vi "Autonomous Independent.vi"() -> ()   [LabVIEW 2018]
doc: "This VI is called when autonomous begins, and will automatically be terminated when autonomous ends. You can carry out timed or sensor driven robot movement independently without needing to return to the caller."
uses:
  <vilib>/Rock Robotics/WPI/DriverStation/WPI_DriverStationDerivedRobotMode.ctl
  <vilib>/Rock Robotics/Network Tables/NT Read String.vi
  Robot Global Data.vi
panel:
  in  "Call Context":T1
  out "Potentiometer":dbl
  out "Yaw":dbl
  out "Right Motor Speed":dbl
  out "Left Motor Speed":dbl
  # "Be sure to right-click and choose Data Operations>>Make Current Value default if you want to save the array values with the VI"
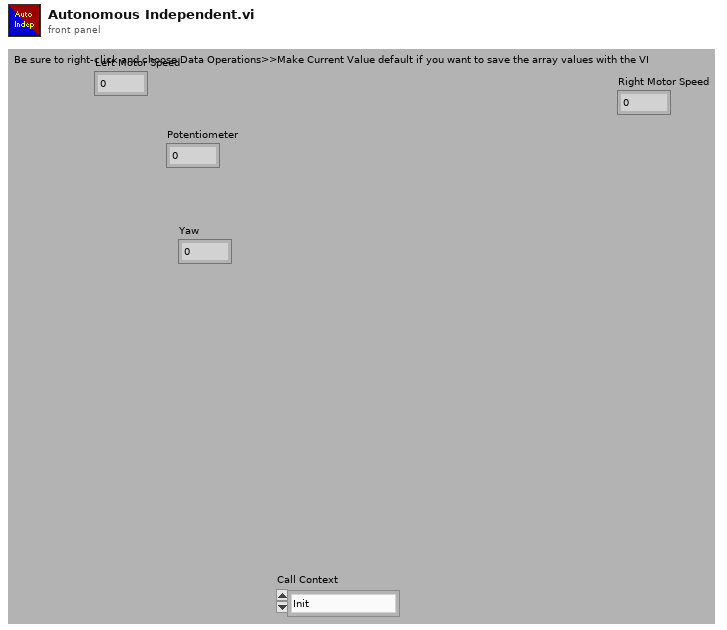
[diagram p1: front panel]
types:
  T1 = typedef "WPI_DriverStationDerivedRobotMode.ctl" = enum16{"Init", "Execute", "Stop"}
  T2 = typedef "WPI_JoystickDevRef.ctl" = cluster{"Device":T3}
  T3 = typedef "WPI_JoystickDeviceEnum.ctl" = enum16{"USB 0", "USB 1", "USB 2", "USB 3", "USB 4", "USB 5"}
  T4 = cluster{"Axes":dbl[], "Buttons":bool[], "POVs":i16[]}
  T5 = cluster{"Yaw":dbl, "Roll":dbl, "Pitch":dbl, "Heading":dbl, "Fused Heading":dbl}
  T6 = typedef "WPI_PotentiometerDevRef.ctl" = cluster{"DevStatus":errorcluster, "Analog Channel":T7, "Invert Output":bool}
  T7 = typedef "FPGA_AIChannel.ctl" = enum8{"AI 0", "AI 1", "AI 2", "AI 3", "AI MXP 0", "AI MXP 1", "AI MXP 2", "AI MXP 3", "Invalid"}
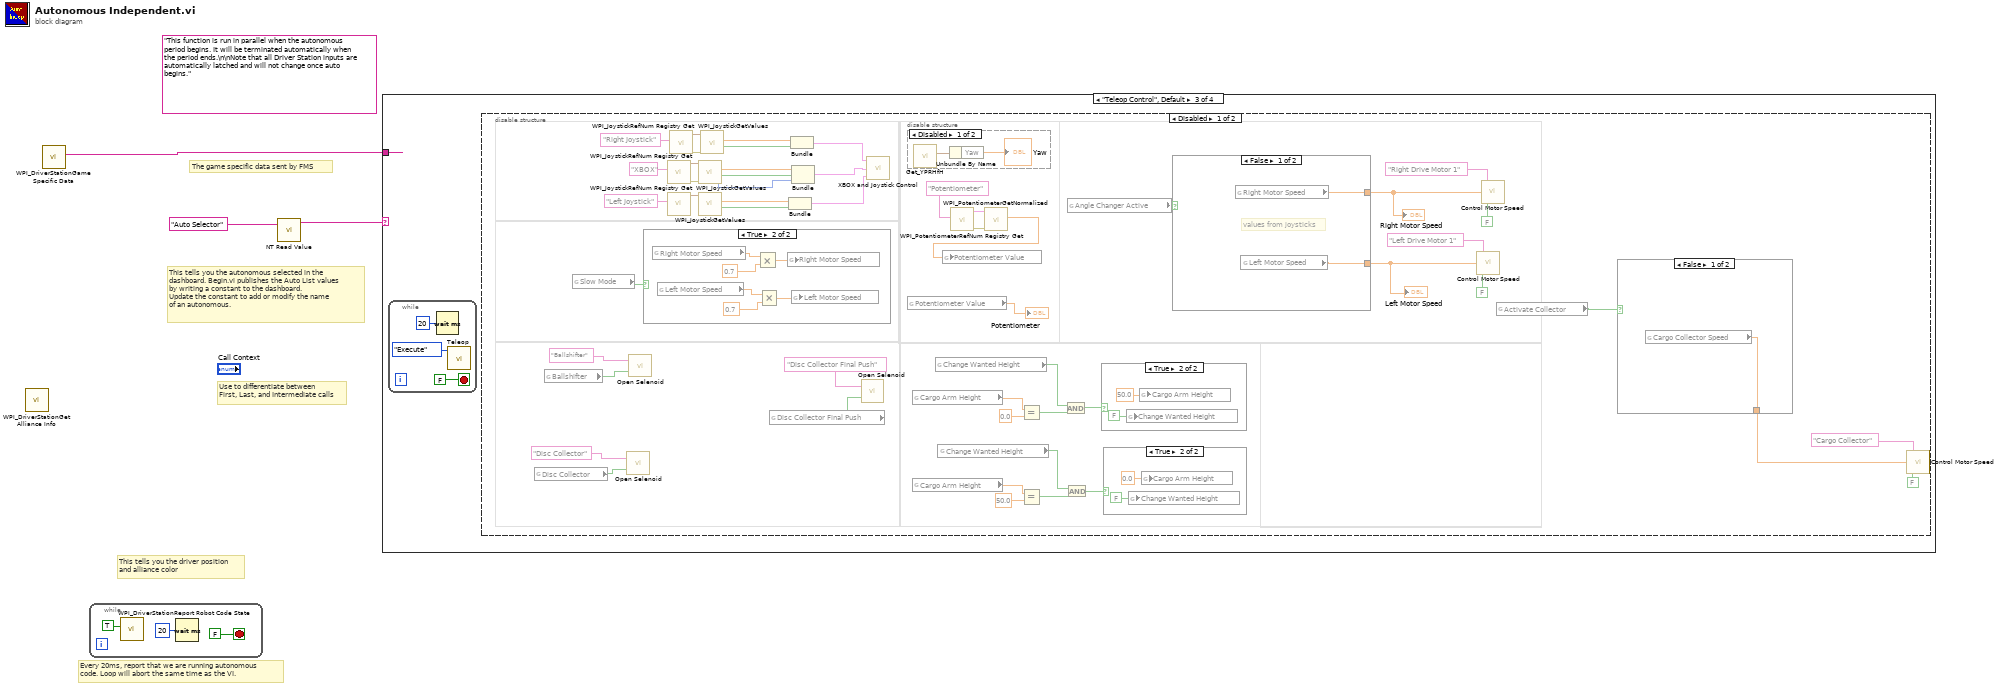
[diagram p0: block diagram]
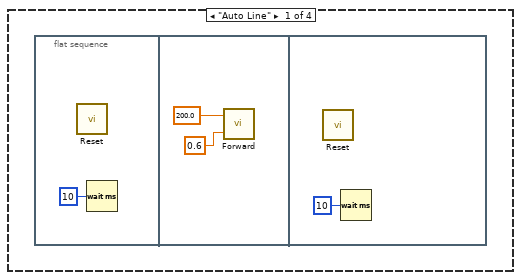
[diagram p2: hidden frame]
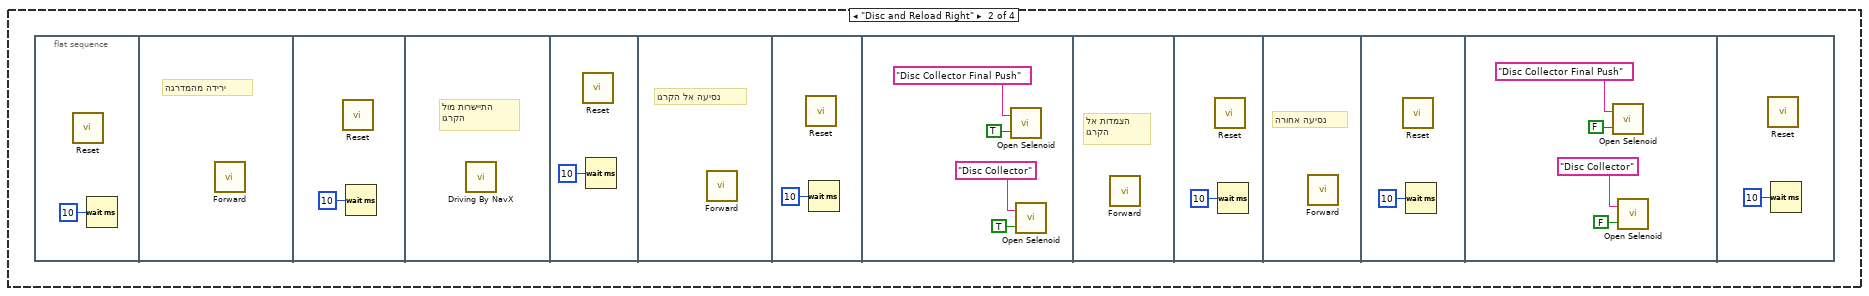
[diagram p3: hidden frame]
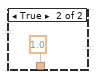
[diagram p4: hidden frame]
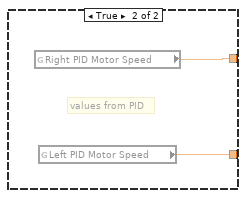
[diagram p6: hidden frame]
diagram:
  (unwired) "This function is run in parallel when the autonomous period begins. It will be terminated automatically when the period ends.\n\nNote that all Driver Station inputs are automatically latched and will not change once auto begins."
  # "Use to differentiate between\nFirst, Last, and Intermediate calls"
  # "The game specific data sent by FMS"
  # "This tells you the autonomous selected in the \ndashboard. Begin.vi publishes the Auto List values\nby writing a constant to the dashboard.\nUpdate the constant to add or modify the name\nof an autonomous."
  # "Every 20ms, report that we are running autonomous\ncode. Loop will abort the same time as the VI."
  # "This tells you the driver position\nand alliance color"
  n1 = call <vilib>:"WPI_DriverStationGet Alliance Info.vi"() -> ()  [unwired: 12 out]
  n2 = call <vilib>:"WPI_DriverStationGame Specific Data.vi"() -> ("Game Specific Data"=w1:string)  [unwired: 11 in]
  n3 = while {
    stop <- FALSE stop-if-true
    n4 = call <vilib>:"WPI_DriverStationReport Robot Code State.vi"("Autonomous"=TRUE) -> ()  [unwired: 10 in, 1 out]
    n5 = Wait (ms)(milliseconds to wait=u32 20) -> ()  [unwired: 1 out]
  }
  n6 = call-poly <vilib>:"NT Read Value.vi"("Name"="Auto Selector") -> ("String"=w2:string)  [unwired: 9 in, 1 out]
  n7 = case shown="\"Teleop Control\", Default" w2 {
    tunnel: w1 -> [_ _ _ _]
    frame "Auto Line" {
      n8 = flat-sequence {
        frame #0 {
          n9 = call "Reset.vi"() -> ()  [unwired: 1 in]
          n10 = Wait (ms)(milliseconds to wait=u32 10) -> ()  [unwired: 1 out]
        }
        frame #1 {
          n11 = call "Forward.vi"("Speed"=0.6, "Driving Distance"=200.0) -> ()  [unwired: 1 in]
        }
        frame #2 {
          n12 = call "Reset.vi"() -> ()  [unwired: 1 in]
          n13 = Wait (ms)(milliseconds to wait=u32 10) -> ()  [unwired: 1 out]
        }
      }
    }
    frame "Disc and Reload Right" {
      n14 = flat-sequence {
        frame #0 {
          n15 = call "Reset.vi"() -> ()  [unwired: 1 in]
          n16 = Wait (ms)(milliseconds to wait=u32 10) -> ()  [unwired: 1 out]
        }
        frame #1 {
          # "ירידה מהמדרגה"
          n17 = call "Forward.vi"() -> ()  [unwired: 3 in]
        }
        frame #2 {
          n18 = call "Reset.vi"() -> ()  [unwired: 1 in]
          n19 = Wait (ms)(milliseconds to wait=u32 10) -> ()  [unwired: 1 out]
        }
        frame #3 {
          # "התיישרות מול\nהקרגו"
          n20 = call "Driving By NavX.vi"() -> ()  [unwired: 4 in]
        }
        frame #4 {
          n21 = call "Reset.vi"() -> ()  [unwired: 1 in]
          n22 = Wait (ms)(milliseconds to wait=u32 10) -> ()  [unwired: 1 out]
        }
        frame #5 {
          # "נסיעה אל הקרגו"
          n23 = call "Forward.vi"() -> ()  [unwired: 3 in]
        }
        frame #6 {
          n24 = call "Reset.vi"() -> ()  [unwired: 1 in]
          n25 = Wait (ms)(milliseconds to wait=u32 10) -> ()  [unwired: 1 out]
        }
        frame #7 {
          n26 = call "Open Selenoid.vi"("Enable"=TRUE, "Selenoid Name"="Disc Collector Final Push") -> ()  [unwired: 1 in]
          n27 = call "Open Selenoid.vi"("Enable"=TRUE, "Selenoid Name"="Disc Collector") -> ()  [unwired: 1 in]
        }
        frame #8 {
          # "הצמדות אל\nהקרגו"
          n28 = call "Forward.vi"() -> ()  [unwired: 3 in]
        }
        frame #9 {
          n29 = call "Reset.vi"() -> ()  [unwired: 1 in]
          n30 = Wait (ms)(milliseconds to wait=u32 10) -> ()  [unwired: 1 out]
        }
        frame #10 {
          # "נסיעה אחורה"
          n31 = call "Forward.vi"() -> ()  [unwired: 3 in]
        }
        frame #11 {
          n32 = call "Reset.vi"() -> ()  [unwired: 1 in]
          n33 = Wait (ms)(milliseconds to wait=u32 10) -> ()  [unwired: 1 out]
        }
        frame #12 {
          n34 = call "Open Selenoid.vi"("Enable"=FALSE, "Selenoid Name"="Disc Collector Final Push") -> ()  [unwired: 1 in]
          n35 = call "Open Selenoid.vi"("Enable"=FALSE, "Selenoid Name"="Disc Collector") -> ()  [unwired: 1 in]
        }
        frame #13 {
          n36 = call "Reset.vi"() -> ()  [unwired: 1 in]
          n37 = Wait (ms)(milliseconds to wait=u32 10) -> ()  [unwired: 1 out]
        }
      }
    }
    frame "Teleop Control", Default {
      n38 = while {
        stop <- FALSE stop-if-true
        n39 = Wait (ms)(milliseconds to wait=u32 20) -> ()  [unwired: 1 out]
        n40 = call "Teleop.vi"("Call Context"=WPI_DriverStationDerivedRobotMode."Execute") -> ()  [unwired: 2 in, 9 out]
      }
      n41 = disable-structure shown="Disabled" {
        frame Disabled {
          n42 = global read "Robot Global Data.vi" "Disc Collector"() -> (w58:bool)
          n43 = global read "Robot Global Data.vi" "Ballshifter"() -> (w60:bool)
          n44 = global read "Robot Global Data.vi" "Slow Mode"() -> (w41:bool)
          n45 = call "Open Selenoid.vi"("Enable"=w58, "Selenoid Name"="Disc Collector") -> ()  [unwired: 1 in]
          n46 = call "Open Selenoid.vi"("Enable"=w60, "Selenoid Name"="Ballshifter") -> ()  [unwired: 1 in]
          n47 = case shown="True" w41 {
            frame False {
            }
            frame True {
              n48 = global read "Robot Global Data.vi" "Right Motor Speed"() -> (w92:dbl)
              n49 = global read "Robot Global Data.vi" "Left Motor Speed"() -> (w89:dbl)
              n50 = Multiply(x=w92, y=0.7) -> (x*y=w91:dbl)
              n51 = Multiply(x=w89, y=0.7) -> (x*y=w88:dbl)
              n52 = global write "Robot Global Data.vi" "Right Motor Speed"(w91) -> ()
              n53 = global write "Robot Global Data.vi" "Left Motor Speed"(w88) -> ()
            }
          }
          n54 = call <vilib>:"WPI_JoystickRefNum Registry Get.vi"("refnum name"="XBOX") -> ("error out"=w79:errorcluster, "JoystickDevRef"=w78:T2)  [unwired: 9 in]
          n55 = call <vilib>:"WPI_JoystickRefNum Registry Get.vi"("refnum name"="Left Joystick") -> ("JoystickDevRef"=w73:T2)  [unwired: 9 in, 1 out]
          n56 = call <vilib>:"WPI_JoystickRefNum Registry Get.vi"("refnum name"="Right Joystick") -> ("error out"=w76:errorcluster, "JoystickDevRef"=w75:T2)  [unwired: 9 in]
          n57 = call <vilib>:"WPI_JoystickGetValues.vi"("error in (no error)"=w79, "JoystickDevRef"=w78) -> ("Buttons"=w68:bool[], "Axes"=w69:dbl[], "POVs"=w37:i16[])  [unwired: 5 in, 2 out]
          n58 = call <vilib>:"WPI_JoystickGetValues.vi"("JoystickDevRef"=w73) -> ("Buttons"=w66:bool[], "Axes"=w70:dbl[])  [unwired: 6 in, 3 out]
          n59 = call <vilib>:"WPI_JoystickGetValues.vi"("error in (no error)"=w76, "JoystickDevRef"=w75) -> ("Buttons"=w71:bool[], "Axes"=w67:dbl[])  [unwired: 5 in, 3 out]
          n60 = global read "Robot Global Data.vi" "Disc Collector Final Push"() -> (w44:bool)
          n61 = Bundle("Axes"=w70, "Buttons"=w66) -> (w64:cluster{"Axes":dbl[], "Buttons":bool[]})  [unwired: 1 in]
          n62 = Bundle("Axes"=w67, "Buttons"=w71) -> (w65:cluster{"Axes":dbl[], "Buttons":bool[]})  [unwired: 1 in]
          n63 = Bundle("Axes"=w69, "Buttons"=w68, "POVs"=w37) -> (w36:T4)  [unwired: 1 in]
          n64 = call "Open Selenoid.vi"("Enable"=w44, "Selenoid Name"="Disc Collector Final Push") -> ()  [unwired: 1 in]
          n65 = call "XBOX and Joystick Control.vi"("Left Joystick"=w64, "XBOX"=w36, "Right Joystick"=w65) -> ()  [unwired: 1 in]
          n66 = disable-structure shown="Disabled" {
            frame Disabled {
              n67 = call <vilib>:"Get_YPRHfH.vi"() -> ("YRPHfH"=w83:T5)  [unwired: 11 in]
              n68 = Unbundle By Name(w83) -> ("Yaw"=→"Yaw":dbl)
            }
            frame Enabled {
            }
          }
          n69 = global read "Robot Global Data.vi" "Potentiometer Value"() -> (→"Potentiometer":dbl)
          n70 = global read "Robot Global Data.vi" "Cargo Arm Height"() -> (w55:dbl)
          n71 = global read "Robot Global Data.vi" "Cargo Arm Height"() -> (w50:dbl)
          n72 = global read "Robot Global Data.vi" "Change Wanted Height"() -> (w52:bool)
          n73 = global read "Robot Global Data.vi" "Change Wanted Height"() -> (w47:bool)
          n74 = call <vilib>:"WPI_PotentiometerRefNum Registry Get.vi"("refnum name"="Potentiometer") -> ("error out"=w35:errorcluster, "PotDevRef"=w34:T6)  [unwired: 9 in]
          n75 = call <vilib>:"WPI_PotentiometerGetNormalized.vi"("error in"=w35, "PotDevRef"=w34) -> ("Normalized Value"=w33:dbl)  [unwired: 7 in, 2 out]
          n76 = global write "Robot Global Data.vi" "Potentiometer Value"(w33) -> ()
          n77 = Equal?(x=w55, y=0.0) -> (x = y?=w53:bool)
          n78 = Equal?(x=w50, y=50.0) -> (x = y?=w48:bool)
          n79 = And(x=w52, y=w53) -> (x .and. y?=w51:bool)
          n80 = And(x=w47, y=w48) -> (x .and. y?=w46:bool)
          n81 = global read "Robot Global Data.vi" "Angle Changer Active"() -> (w38:bool)
          n82 = case shown="True" w51 {
            frame False {
            }
            frame True {
              n83 = global write "Robot Global Data.vi" "Change Wanted Height"(FALSE ("Change Wanted Height")) -> ()
              n84 = global write "Robot Global Data.vi" "Cargo Arm Height"(50.0 ("Cargo Arm Height")) -> ()
            }
          }
          n85 = case shown="True" w46 {
            frame False {
            }
            frame True {
              n86 = global write "Robot Global Data.vi" "Change Wanted Height"(FALSE ("Change Wanted Height")) -> ()
              n87 = global write "Robot Global Data.vi" "Cargo Arm Height"(0.0 ("Cargo Arm Height")) -> ()
            }
          }
          n88 = case shown="False" w38 {
            tunnel: [w85 w87] -> w40
            tunnel: [w84 w86] -> w39
            frame False {
              # "values from joysticks"
              n89 = global read "Robot Global Data.vi" "Right Motor Speed"() -> (w85:dbl)
              n90 = global read "Robot Global Data.vi" "Left Motor Speed"() -> (w84:dbl)
            }
            frame True {
              # "values from PID"
              n91 = global read "Robot Global Data.vi" "Right PID Motor Speed"() -> (w87:dbl)
              n92 = global read "Robot Global Data.vi" "Left PID Motor Speed"() -> (w86:dbl)
            }
          }
          "Left Motor Speed" <- w39
          "Right Motor Speed" <- w40
          n93 = call "Control Motor Speed.vi"("Invert"=FALSE, "Speed"=w39, "Motor Name"="Left Drive Motor 1") -> ()  [unwired: 1 in]
          n94 = call "Control Motor Speed.vi"("Invert"=FALSE, "Speed"=w40, "Motor Name"="Right Drive Motor 1") -> ()  [unwired: 1 in]
          n95 = global read "Robot Global Data.vi" "Activate Collector"() -> (w30:bool)
          n96 = case shown="False" w30 {
            tunnel: [w80 1.0 ("Cargo Collector Speed")] -> w29
            frame False {
              n97 = global read "Robot Global Data.vi" "Cargo Collector Speed"() -> (w80:dbl)
            }
            frame True {
            }
          }
          n98 = call "Control Motor Speed.vi"("Invert"=FALSE, "Speed"=w29, "Motor Name"="Cargo Collector") -> ()  [unwired: 1 in]
        }
        frame Enabled {
        }
      }
    }
    frame "Nothing" {
    }
  }
